vi "Measure Frequency.vi"(0 "Waveform":waveform(dbl)={"t0"=timestamp(0 s since 1904-01-01), "dt"=0.0, "Y"=[]}, 11 "error in":errorcluster) -> (4 "exported spectrum (dB)":T1 {"dB Spectrum (Hann)" format="%.2f"; "df" format="%.2f"; "f0" format="%.2f"}, 6 "frequency":dbl format="%.2f", 8 "Vpeak":dbl format="%.2p", 15 "error out":errorcluster)   [LabVIEW 2012]
uses:
  <vilib>/measure/matone.llb/Extract Single Tone Information 1 Chan.vi
  <vilib>/measure/NI_MAPro.lvlib
panel:
  in  "advanced search":T2={"approx freq. (optional)"=1544000.0, "search (+/- % of Fsampl.)"=0.1} {"search (+/- % of Fsampl.)" format="%.2p"; "approx freq. (optional)" format="%.4p"}
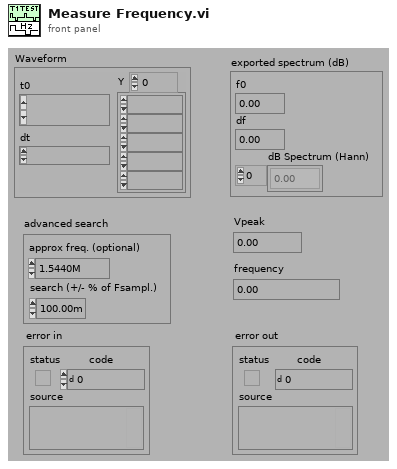
[diagram p1: front panel]
types:
  T1 = cluster{"f0":dbl, "df":dbl, "dB Spectrum (Hann)":dbl[]}
  T2 = cluster{"approx freq. (optional)":dbl, "search (+/- % of Fsampl.)":dbl}
  T3 = enum16{"none", "input signal", "detected signal", "residual signal"}
  T4 = cluster{"exported time signal":waveform(dbl), "exported spectrum (dB)":cluster{"f0":dbl, "df":dbl, "dB Spectrum (Hann)":dbl[]}}
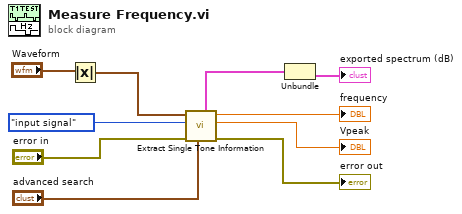
[diagram p0: block diagram]
diagram:
  n1 = Absolute Value(x="Waveform") -> (abs(x)=w9:waveform(dbl))
  n2 = call-poly <vilib>:"Extract Single Tone Information.vi"("advanced search"="advanced search", "error in (no error)"="error in", "export mode"=T3."input signal" ("export signals"), "time signal in"=w9) -> ("error out"=→"error out":errorcluster, "detected amplitude"=→"Vpeak":dbl, "detected frequency"=→"frequency":dbl, "exported signals"=w6:T4)  [unwired: 2 in, 2 out]
  n3 = Unbundle(w6) -> ("exported spectrum (dB)"=→"exported spectrum (dB)":T1)  [unwired: 1 out]
